vi "GenerateOverriddenSystemDefinition.vi"(8 "error in (no error)":errorcluster, 10 "absolute configuration files":path[](array[path]), 11 "absolute system definition file":path) -> (0 "error out":errorcluster, 1 "Temporary File?":bool, 2 "properties":T1[](array[typedef]), 3 "absolute overridden system definition file":path)   [LabVIEW 2017, in "VeriStandTestUtilities.lvlib"]
uses:
  VeriStandTestUtilities.lvlib
  ConfigPropertyItem.ctl
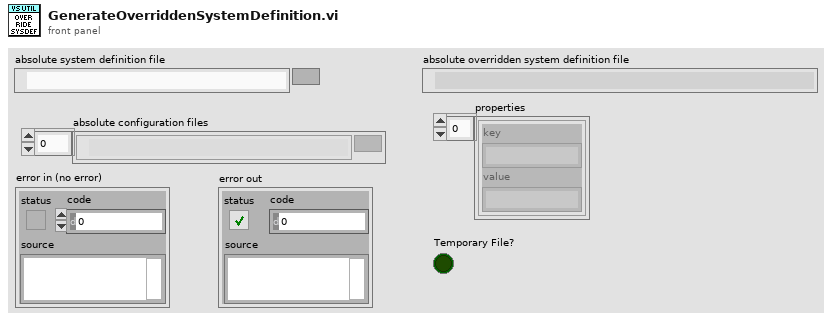
[diagram p1: front panel]
types:
  T1 = typedef "VeriStandTestUtilities.lvlib/ConfigPropertyItem.ctl" = cluster{"key":string, "value":string}
  T2 = typedef "VeriStandTestUtilities.lvlib/ConfigOverrideItem.ctl" = cluster{"node":string, "property":string, "value":string}
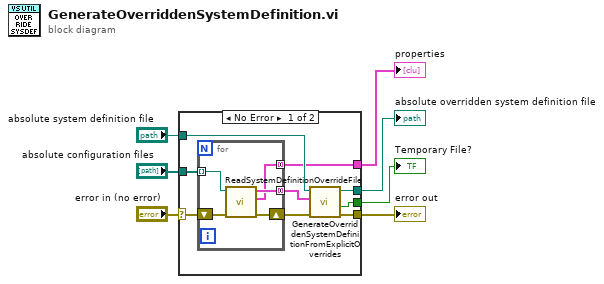
[diagram p0: block diagram]
diagram:
  n1 = case shown="No Error" "error in (no error)" {
    selector: "error in (no error)" -> [w12 w23]
    tunnel: "absolute configuration files" -> [w15 _]
    tunnel: "absolute system definition file" -> [w16 w22]
    tunnel: [w10 w23] -> w4
    tunnel: [w9 w22] -> w3
    tunnel: [w14 _] -> w2
    tunnel: [w8 _] -> w1
    frame No Error {
      n2 = for {
        shift-right: [w20] -> w11
        shift-left: w12 -> [w21]
        tunnel: w15 -> [w19] mode=indexing
        tunnel: [w18] -> w13 mode=concatenating
        tunnel: [w17] -> w14 mode=concatenating
        n3 = call "ReadSystemDefinitionOverrideFile.vi"("error in (no error)"=w21, "configuration file path"=w19) -> ("error out"=w20:errorcluster, "properties"=w17:T1[], "overrides"=w18:T2[])  [unwired: 7 in]
      }
      n4 = call "GenerateOverriddenSystemDefinitionFromExplicitOverrides.vi"("error in (no error)"=w11, "overrides"=w13, "absolute system definition file"=w16) -> ("error out"=w10:errorcluster, "Temporary File?"=w8:bool, "absolute overridden system definition file"=w9:path)  [unwired: 6 in]
    }
    frame Error {
    }
  }
  "error out" <- w4
  "absolute overridden system definition file" <- w3
  "properties" <- w2
  "Temporary File?" <- w1
